vi "Read Tester Tx.vi"(8 "error in (no error)":errorcluster, 11 "Panel in":refnum<class "Station Actor.lvclass">) -> (0 "error out":errorcluster, 3 "Panel out":refnum<class "Station Actor.lvclass">)   [LabVIEW 2019, in "Station Actor.lvlib" / "Station Actor.lvclass"]
uses:
  Station Actor.lvclass
  Station Actor.lvclass/Station Actor.ctl
  <vilib>/OPCUA/server/Read Variant.vi
  <vilib>/OPCUA/NI OPC UA Server.lvlib
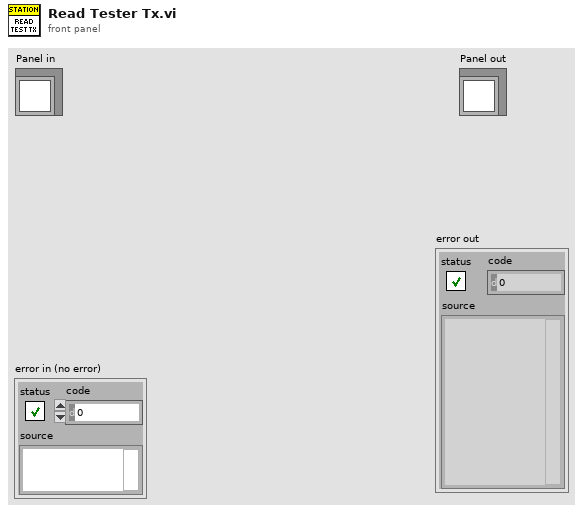
[diagram p1: front panel]
types:
  T1 = typedef "OPC UA Server Refnum.ctl" = refnum<k21>
  T2 = typedef "NodeId.ctl" = string
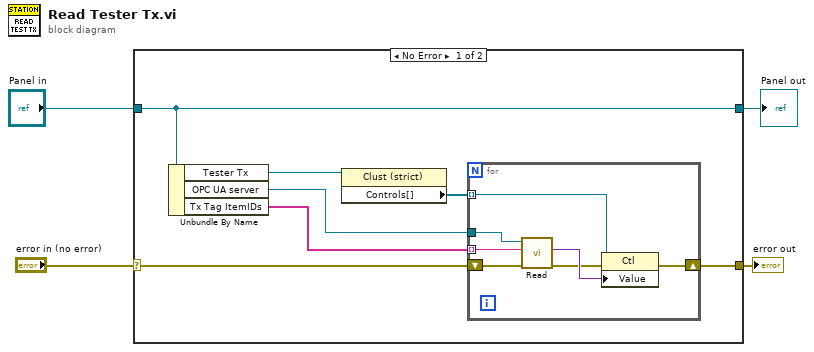
[diagram p0: block diagram]
diagram:
  n1 = case shown="No Error" "error in (no error)" {
    selector: "error in (no error)" -> [w7 w20]
    tunnel: [w6 w20] -> w3
    tunnel: [w8 w19] -> w1
    tunnel: "Panel in" -> [w8 w19]
    frame No Error {
      n2 = Unbundle By Name(w8) -> ("Tester Tx"=w5:refnum<vi>, "OPC UA server"=w10:T1, "Tx Tag ItemIDs"=w11:T2[])
      n3 = property class="Clust (strict)"(reference=w5) -> ("Controls[]"=w9:refnum<vi>[])  [unwired: 1 in, 2 out]
      n4 = for {
        tunnel: w10 -> [w18]
        tunnel: w11 -> [w16] mode=indexing
        shift-right: [w12] -> w6
        shift-left: w7 -> [w17]
        tunnel: w9 -> [w15] mode=indexing
        n5 = call-poly <vilib>:"Read.vi"("error in (no error)"=w17, "node ID"=w16, "OPC UA server refnum in"=w18) -> ("error out"=w13:errorcluster, "value"=w14:variant)  [unwired: 4 in, 3 out]
        n6 = property class="Ctl"(reference=w15, error in=w13, "Value"=w14) -> (error out=w12:errorcluster)  [unwired: 1 out]
      }
    }
    frame Error {
    }
  }
  "error out" <- w3
  "Panel out" <- w1
